vi "Corr2Coef IMAQ U16.vi"(0 "Image A":T1, 7 "Image B":T1, 11 "Error In":errorcluster) -> (8 "Corr Coef":dbl, 15 "Error Out":errorcluster)   [LabVIEW 2020]
uses:
  <vilib>/vision/Image Controls.llb/IMAQ Image.ctl
  <vilib>/vision/NI_Vision_Development_Module.lvlib
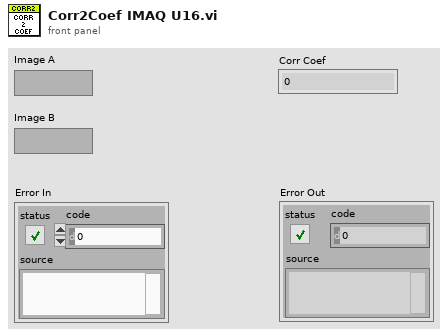
[diagram p1: front panel]
types:
  T1 = typedef "IMAQ Image.ctl" = refnum<image>
  T2 = cluster{"Mean Value":sgl, "Standard Variation":sgl, "Minimal Value":sgl, "Maximal Value":sgl, "Area (calibrated)":sgl, "Area (pixels)":u32, "%":sgl, "Calibration Valid":bool}
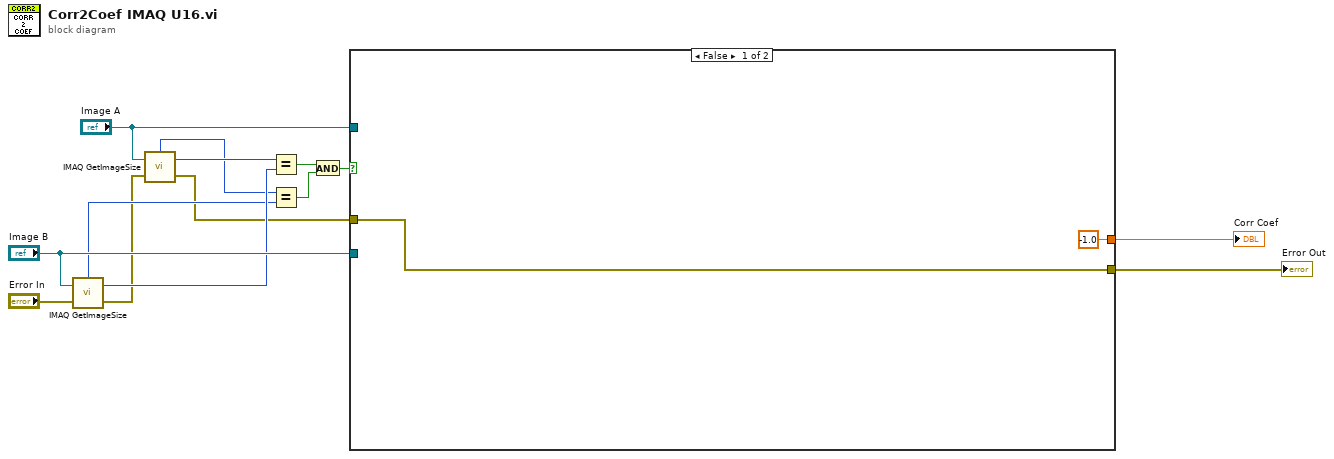
[diagram p0: block diagram]
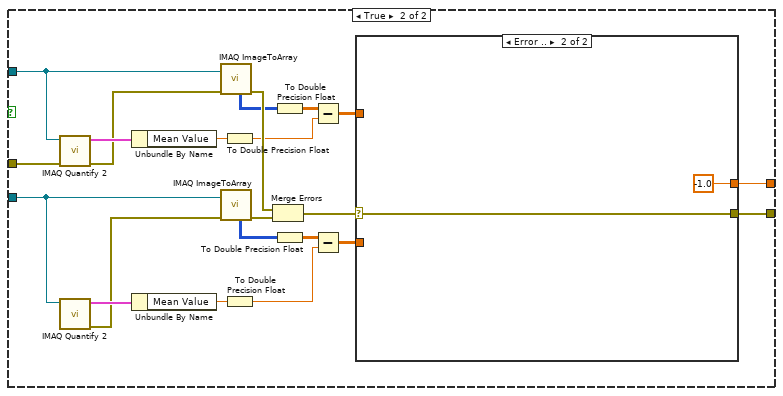
[diagram p2: hidden frame]
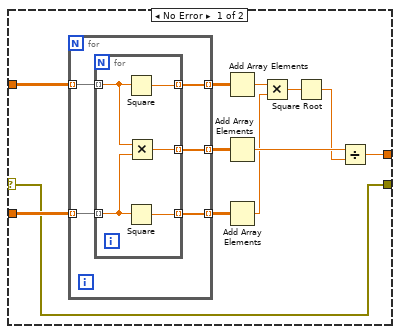
[diagram p3: hidden frame]
diagram:
  n1 = call "IMAQ GetImageSize"("Image"="Image B", "error in (no error)"="Error In") -> ("Y Resolution"=w9:i32, "X Resolution"=w7:i32, "error out"=w2:errorcluster)  [unwired: 2 in]
  n2 = call "IMAQ GetImageSize"("Image"="Image A", "error in (no error)"=w2) -> ("Y Resolution"=w10:i32, "X Resolution"=w8:i32, "error out"=w4:errorcluster)  [unwired: 2 in]
  n3 = Equal?(x=w10, y=w9) -> (x = y?=w6:bool)
  n4 = Equal?(x=w8, y=w7) -> (x = y?=w5:bool)
  n5 = And(x=w6, y=w5) -> (x .and. y?=w1:bool)
  n6 = case shown="False" w1 {
    tunnel: [-1.0 w31] -> w14
    tunnel: [w15 w22] -> w13
    tunnel: "Image A" -> [_ w19]
    tunnel: "Image B" -> [_ w18]
    tunnel: w4 -> [w15 w17]
    frame False {
    }
    frame True {
      n7 = call "IMAQ Quantify 2"("error in (no error)"=w17, "Image"=w19) -> ("error out"=w23:errorcluster, "Global Report"=w38:T2)  [unwired: 7 in, 1 out]
      n8 = call "IMAQ Quantify 2"("Image"=w18) -> ("error out"=w24:errorcluster, "Global Report"=w35:T2)  [unwired: 8 in, 1 out]
      n9 = Unbundle By Name(w38) -> ("Mean Value"=w37:sgl)
      n10 = Unbundle By Name(w35) -> ("Mean Value"=w36:sgl)
      n11 = call "IMAQ ImageToArray"("error in (no error)"=w23, "Image"=w19) -> ("Image Pixels (U16)"=w21:u16[][], "error out"=w34:errorcluster)  [unwired: 2 in, 3 out]
      n12 = call "IMAQ ImageToArray"("error in (no error)"=w24, "Image"=w18) -> ("Image Pixels (U16)"=w20:u16[][], "error out"=w33:errorcluster)  [unwired: 2 in, 3 out]
      n13 = To Double Precision Float(number=w37) -> (double precision float=w25:dbl)
      n14 = To Double Precision Float(number=w36) -> (double precision float=w26:dbl)
      n15 = Merge Errors(w34, w33) -> (w32:errorcluster)
      n16 = To Double Precision Float(number=w21) -> (double precision float=w30:dbl[][])
      n17 = To Double Precision Float(number=w20) -> (double precision float=w29:dbl[][])
      n18 = Subtract(x=w30, y=w25) -> (x-y=w28:dbl[][])
      n19 = Subtract(x=w29, y=w26) -> (x-y=w27:dbl[][])
      n20 = case shown="Error .." w32 {
        selector: w32 -> [w39 w61]
        tunnel: [w42 -1.0] -> w31
        tunnel: w28 -> [w41 _]
        tunnel: w27 -> [w40 _]
        tunnel: [w39 w61] -> w22
        frame No Error {
          n21 = for {
            tunnel: w41 -> [w55] mode=indexing
            tunnel: w40 -> [w54] mode=indexing
            tunnel: [w53] -> w50 mode=indexing
            tunnel: [w52] -> w48 mode=indexing
            tunnel: [w51] -> w49 mode=indexing
            n22 = for {
              tunnel: w55 -> [w60] mode=indexing
              tunnel: w54 -> [w59] mode=indexing
              tunnel: [w58] -> w53 mode=indexing
              tunnel: [w57] -> w52 mode=indexing
              tunnel: [w56] -> w51 mode=indexing
              n23 = Square(x=w60) -> (x^2=w58:dbl)
              n24 = Square(x=w59) -> (x^2=w56:dbl)
              n25 = Multiply(x=w60, y=w59) -> (x*y=w57:dbl)
            }
          }
          n26 = Add Array Elements(numeric array=w50) -> (sum=w46:dbl)
          n27 = Add Array Elements(numeric array=w48) -> (sum=w47:dbl)
          n28 = Add Array Elements(numeric array=w49) -> (sum=w45:dbl)
          n29 = Multiply(x=w46, y=w45) -> (x*y=w44:dbl)
          n30 = Square Root(x=w44) -> (sqrt(x)=w43:dbl)
          n31 = Divide(x=w47, y=w43) -> (x/y=w42:dbl)
        }
        frame Error {
        }
      }
    }
  }
  "Corr Coef" <- w14
  "Error Out" <- w13
